vi "条件结构的使用(上).vi"() -> ()   [LabVIEW 2018]
panel:
  out "数值":dbl
  in  "下拉列表 2":u16(ring) items=["x/y", "x*y", "x-y", "x+y"]
  in  "y":dbl
  in  "x":dbl
  out "输出":string
  in  "下拉列表":u16(ring) items=["我要自学网", "51自学网", "51zxw", "第四种状态"]
  out "滑动杆":dbl(slide) scale=0.0..10.0
  in  "布尔":bool
  in  "停止":bool
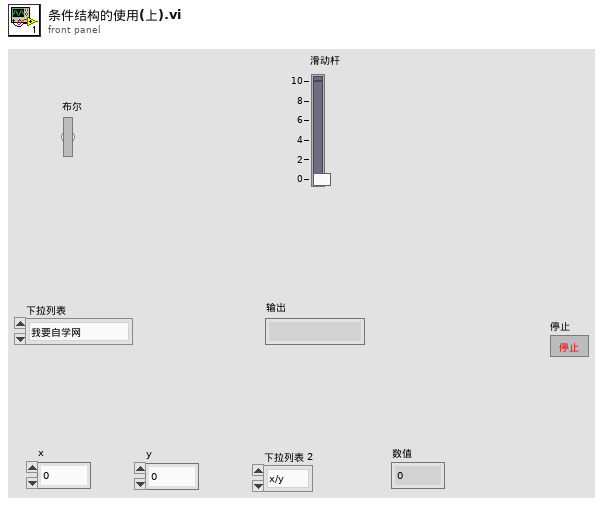
[diagram p1: front panel]
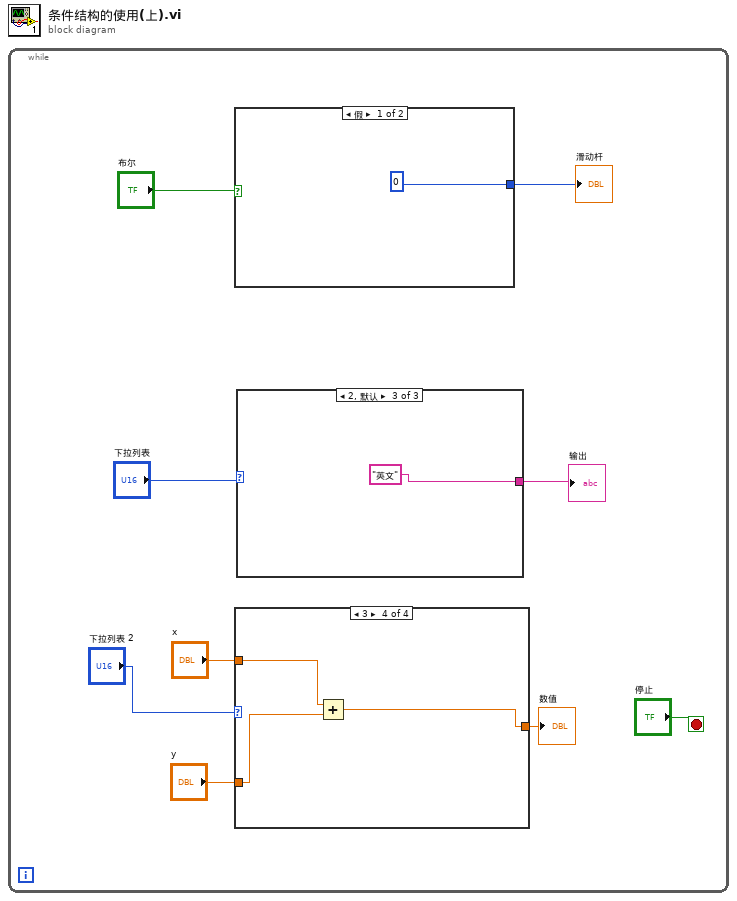
[diagram p0: block diagram]
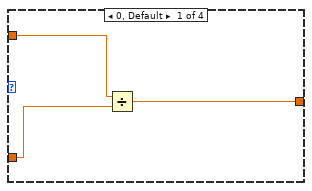
[diagram p2: hidden frame]
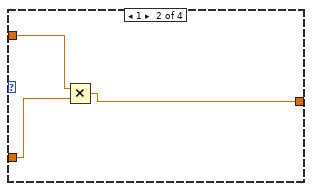
[diagram p3: hidden frame]
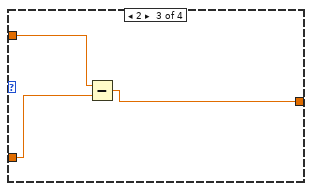
[diagram p4: hidden frame]
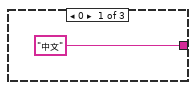
[diagram p5: hidden frame]
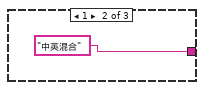
[diagram p6: hidden frame]
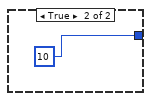
[diagram p7: hidden frame]
diagram:
  n1 = while {
    stop <- "停止" stop-if-true
    n2 = case shown="假" "布尔" {
      tunnel: [0 10] -> w7
      frame False {
      }
      frame True {
      }
    }
    "滑动杆" <- w7
    n3 = case shown="3" "下拉列表 2" {
      tunnel: "x" -> [w11 w14 w18 w20]
      tunnel: "y" -> [w12 w15 w17 w21]
      tunnel: [w10 w13 w16 w19] -> w1
      frame 0, Default {
        n4 = Divide(x=w11, y=w12) -> (x/y=w10:dbl)
      }
      frame 1 {
        n5 = Multiply(x=w14, y=w15) -> (x*y=w13:dbl)
      }
      frame 2 {
        n6 = Subtract(x=w18, y=w17) -> (x-y=w16:dbl)
      }
      frame 3 {
        n7 = Add(x=w20, y=w21) -> (x+y=w19:dbl)
      }
    }
    "数值" <- w1
    n8 = case shown="2, 默认" "下拉列表" {
      tunnel: ["中文" "中英混合" "英文"] -> w5
      frame 0 {
      }
      frame 1 {
      }
      frame 2, Default {
      }
    }
    "输出" <- w5
  }
